vi "ConfigInputLoopEnd.vi"(1 "MulticolumnListbox in":refnum<vi>, 2 "ID":u8, 3 "ItemNames in":string[][](array[string])) -> (0 "ItemNames out":string[][](array[string]))   [LabVIEW 2018, in "Config.lvlib"]
uses:
  Config.lvlib
panel:
  in  "Replace":bool
  in  "Insert":bool
  in  "Append":bool
  # "Loop End"
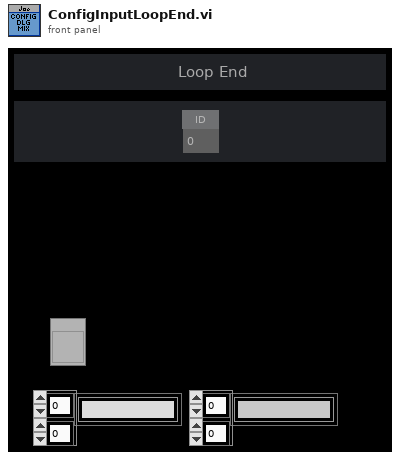
[diagram p1: front panel]
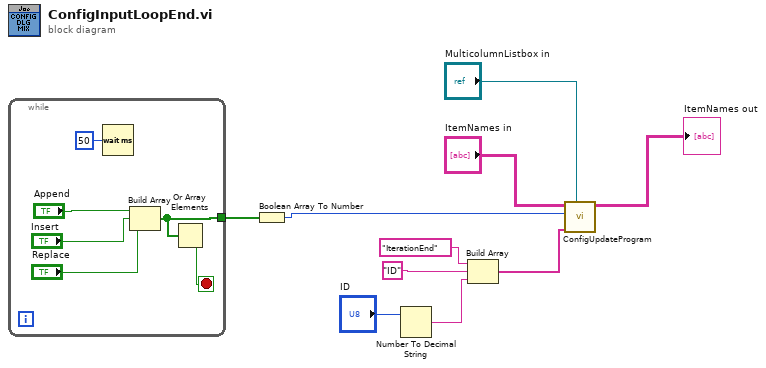
[diagram p0: block diagram]
diagram:
  n1 = while {
    tunnel: [w12] -> w10
    stop <- w13 stop-if-true
    n2 = Wait (ms)(milliseconds to wait=u32 50) -> ()  [unwired: 1 out]
    n3 = Build Array("Append", "Insert", "Replace") -> (w12:bool[])
    n4 = Or Array Elements(Boolean array=w12) -> (logical OR=w13:bool)
  }
  n5 = Boolean Array To Number(Boolean array=w10) -> (number=w9:u32)
  n6 = Number To Decimal String(number="ID") -> (decimal integer string=w3:string)  [unwired: 1 in]
  n7 = Build Array("IterationEnd", "ID" ("element"), w3) -> (w1:string[])
  n8 = call "ConfigUpdateProgram.vi"("MulticolumnListbox in"="MulticolumnListbox in", "New Element"=w1, "Operation"=w9, "ItemNames in"="ItemNames in") -> ("ItemNames out"=→"ItemNames out":string[][])  [unwired: 7 in]
